vi "change.vi"(6 "dark":u8, 7 "white":u8, 9 "lie":u32, 10 "hang":u32, 11 "a":u32[](array[numeric])=[0, 0, 0, 0, 0, 0, 0, 0, 0, 0, 0, 0, 0, 0, 0, 0, 0, 0, 0, 0, 0, 0, 0, 0, 0, 0, 0, 0, 0, 0, 0, 0, 0, 0, 0, 0, 0, 0, 0, 0, 0, 0, 0, 0, 0, 0, 0, 0, 0, 0, 0, 0, 0, 0, 0, 0, 0, 0, 0, 0, 0, 0, 0, 0, 0, 0, 0, 0, 0, 0, 0, 0, 0, 0, 0, 0, 0, 0, 0, 0, 0, 0, 0, 0, 0, 0, 0, 0, 0, 0, 0, 0, 0, 0, 0, 0, 0, 0, 0, 0, 0, 0, 0, 0, 0, 0, 0, 0, 0, 0, 0, 0, 0, 0, 0, 0, 0, 0, 0, 0, 0, 0, 0, 0, 0, 0, 0, 0, 0, 0]) -> (3 "a out":u32[](array[numeric]))   [LabVIEW 2014, in "test.lvlib"]
doc: "__declspec( dllexport ) void change(unsigned int a[X_MAX][Y_MAX], unsigned int hang, unsigned int lie,unsigned char white,unsigned char dark);"
uses:
  test.lvlib
  test/Debug/test.dll
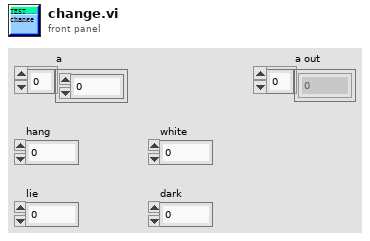
[diagram p1: front panel]
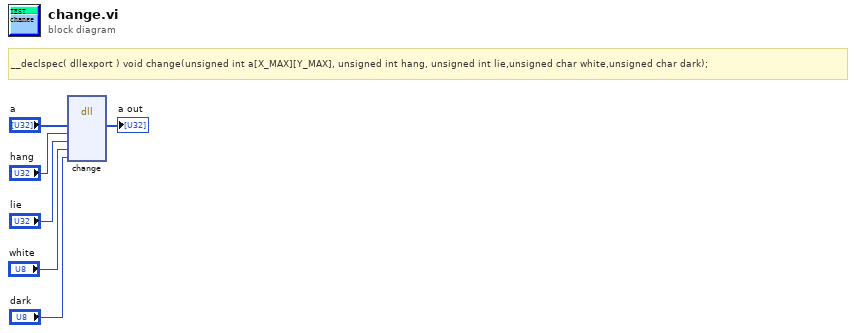
[diagram p0: block diagram]
diagram:
  # "__declspec( dllexport ) void\tchange(unsigned int a[X_MAX][Y_MAX], unsigned int hang, unsigned int lie,unsigned char white,unsigned char dark);"
  n1 = dll-call lib="PTH2Cabs CUsers\tlove  benDesktopNI项目testDebugtest.*" fn="change"("a"="a", "hang"="hang", "lie"="lie", "white"="white", "dark"="dark") -> ("a"=→"a out":u32[])  [unwired: 8 in, 2 out]
